vi "GetLibIconForVIIconOverlay.vi"(11 "Library":refnum<vi>) -> (2 "Library Icon For VI Overlay":T1 {"Rectangle"."bottom" min=0 max=0; "Rectangle"."right" min=0 max=0; "Rectangle"."top" min=0 max=0; "Rectangle"."left" min=0 max=0; "colors" max=0; "mask" max=0; "image" max=0; "image depth" min=0 max=0; "image type" min=0 max=0})   [LabVIEW 2020]
uses:
  <vilib>/picture/picture.llb/imagedata.ctl
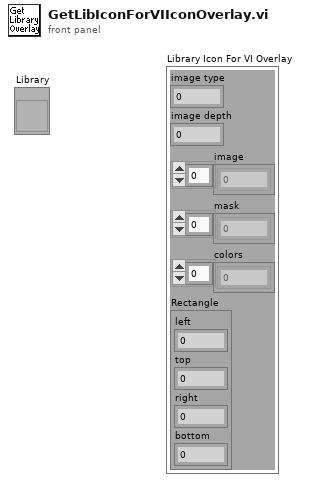
[diagram p1: front panel]
types:
  T1 = typedef "imagedata.ctl" = cluster{"image type":i32, "image depth":i32, "image":u8[], "mask":u8[], "colors":u32[], "Rectangle":cluster{"left":i16, "top":i16, "right":i16, "bottom":i16}}
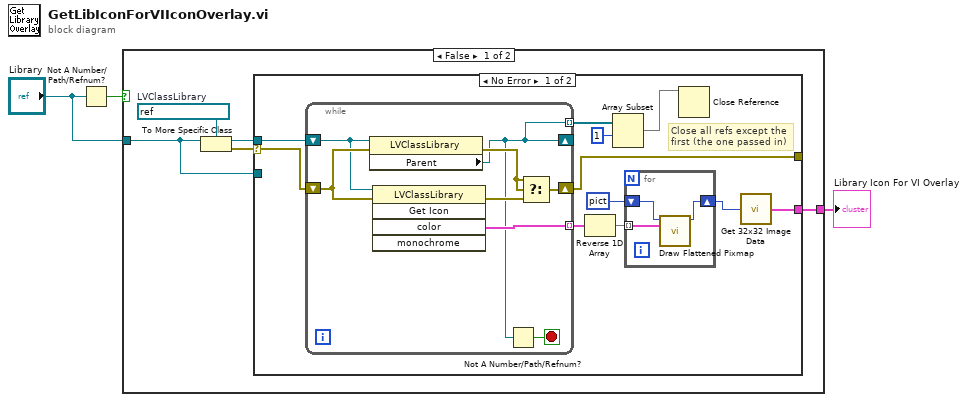
[diagram p0: block diagram]
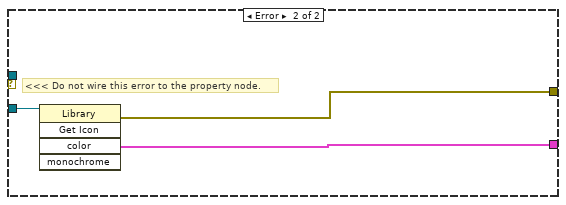
[diagram p2: hidden frame]
diagram:
  n1 = Not A Number/Path/Refnum?(number/path/refnum="Library") -> (NaN/Path/Refnum?=w3:bool)
  n2 = case shown="False" w3 {
    tunnel: "Library" -> [w5 _]
    tunnel: [w4 _] -> w2
    frame False {
      w8 = refnum<vi> refnum  # LVClassLibrary
      n3 = To More Specific Class(target class=w8, reference=w5) -> (specific class reference=w6:refnum<vi>, error out=w7:errorcluster)  [unwired: 1 in]
      n4 = case shown="No Error" w7 {
        selector: w7 -> [w12 _]
        tunnel: w6 -> [w19 _]
        tunnel: [w15 w33] -> w4
        tunnel: [w13 w32] -> _
        tunnel: w5 -> [_ w31]
        frame No Error {
          # "Close all refs except the\nfirst (the one passed in)"
          n5 = while {
            shift-right: [w24] -> _
            shift-left: w19 -> [w23]
            shift-right: [w26] -> w13
            shift-left: w12 -> [w29]
            tunnel: [w25] -> w18 mode=indexing
            tunnel: [w24] -> w11 mode=indexing
            stop <- w30 stop-if-true
            n6 = property class="LVClassLibrary"(reference=w23, error in=w29) -> (error out=w28:errorcluster, "Parent"=w24:refnum<vi>)  [unwired: 1 out]
            n7 = invoke class="LVClassLibrary" method="Get Icon"(reference=w23, error in=w29) -> (error out=w27:errorcluster, "color"=w25:T1)  [unwired: 3 in, 3 out]
            n8 = Not A Number/Path/Refnum?(number/path/refnum=w24) -> (NaN/Path/Refnum?=w30:bool)
            n9 = Select(t=w28, s=w28, f=w27) -> (s? t:f=w26:errorcluster)
          }
          n10 = Reverse 1D Array(array=w18) -> (reversed array=w17:T1[])
          n11 = Array Subset(array=w11, index=1) -> (w9:refnum<vi>[])  [unwired: 1 in]
          n12 = for {
            tunnel: w17 -> [w22] mode=indexing
            shift-right: [w21] -> w14
            shift-left: picture data[5B] ("new picture") -> [w20]
            n13 = call <vilib>:"Draw Flattened Pixmap.vi"("image data"=w22, "picture"=w20) -> ("new picture"=w21:picture)  [unwired: 7 out]
          }
          n14 = Close Reference(reference=w9) -> ()  [unwired: 1 in, 1 out]
          n15 = call "Get 32x32 Image Data.vi"("new picture"=w14) -> ("image data"=w15:T1)
        }
        frame Error {
          # "<<< Do not wire this error to the property node."
          n16 = invoke class="Library" method="Get Icon"(reference=w31) -> (error out=w32:errorcluster, "color"=w33:T1)  [unwired: 4 in, 3 out]
        }
      }
    }
    frame True {
    }
  }
  "Library Icon For VI Overlay" <- w2
